vi "SubGenCodeRobot.vi"(8 "Edge Right Side":cluster{cluster{"Xrn":dbl, "Yrn":dbl}}[](array[cluster]), 11 "Edge Left Side":cluster{cluster{"Xln":dbl, "Yln":dbl}}[](array[cluster])) -> (3 "Source CODE Robot":string)   [LabVIEW 2015]
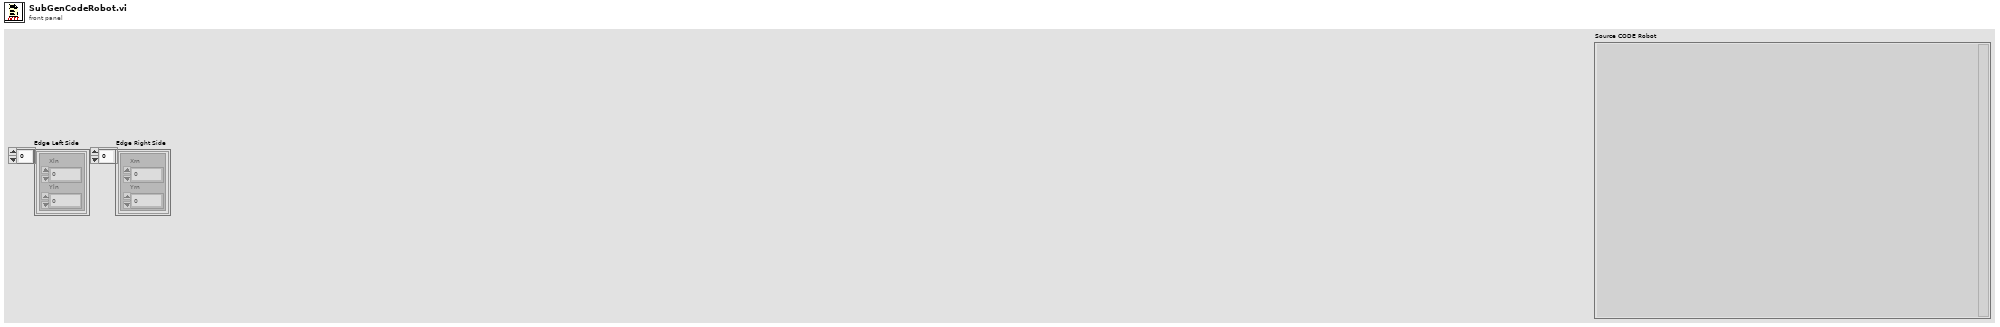
[diagram p1: front panel]
types:
  T1 = enum16{"open", "replace", "create", "open or create", "replace or create", "replace or create with confirmation"}
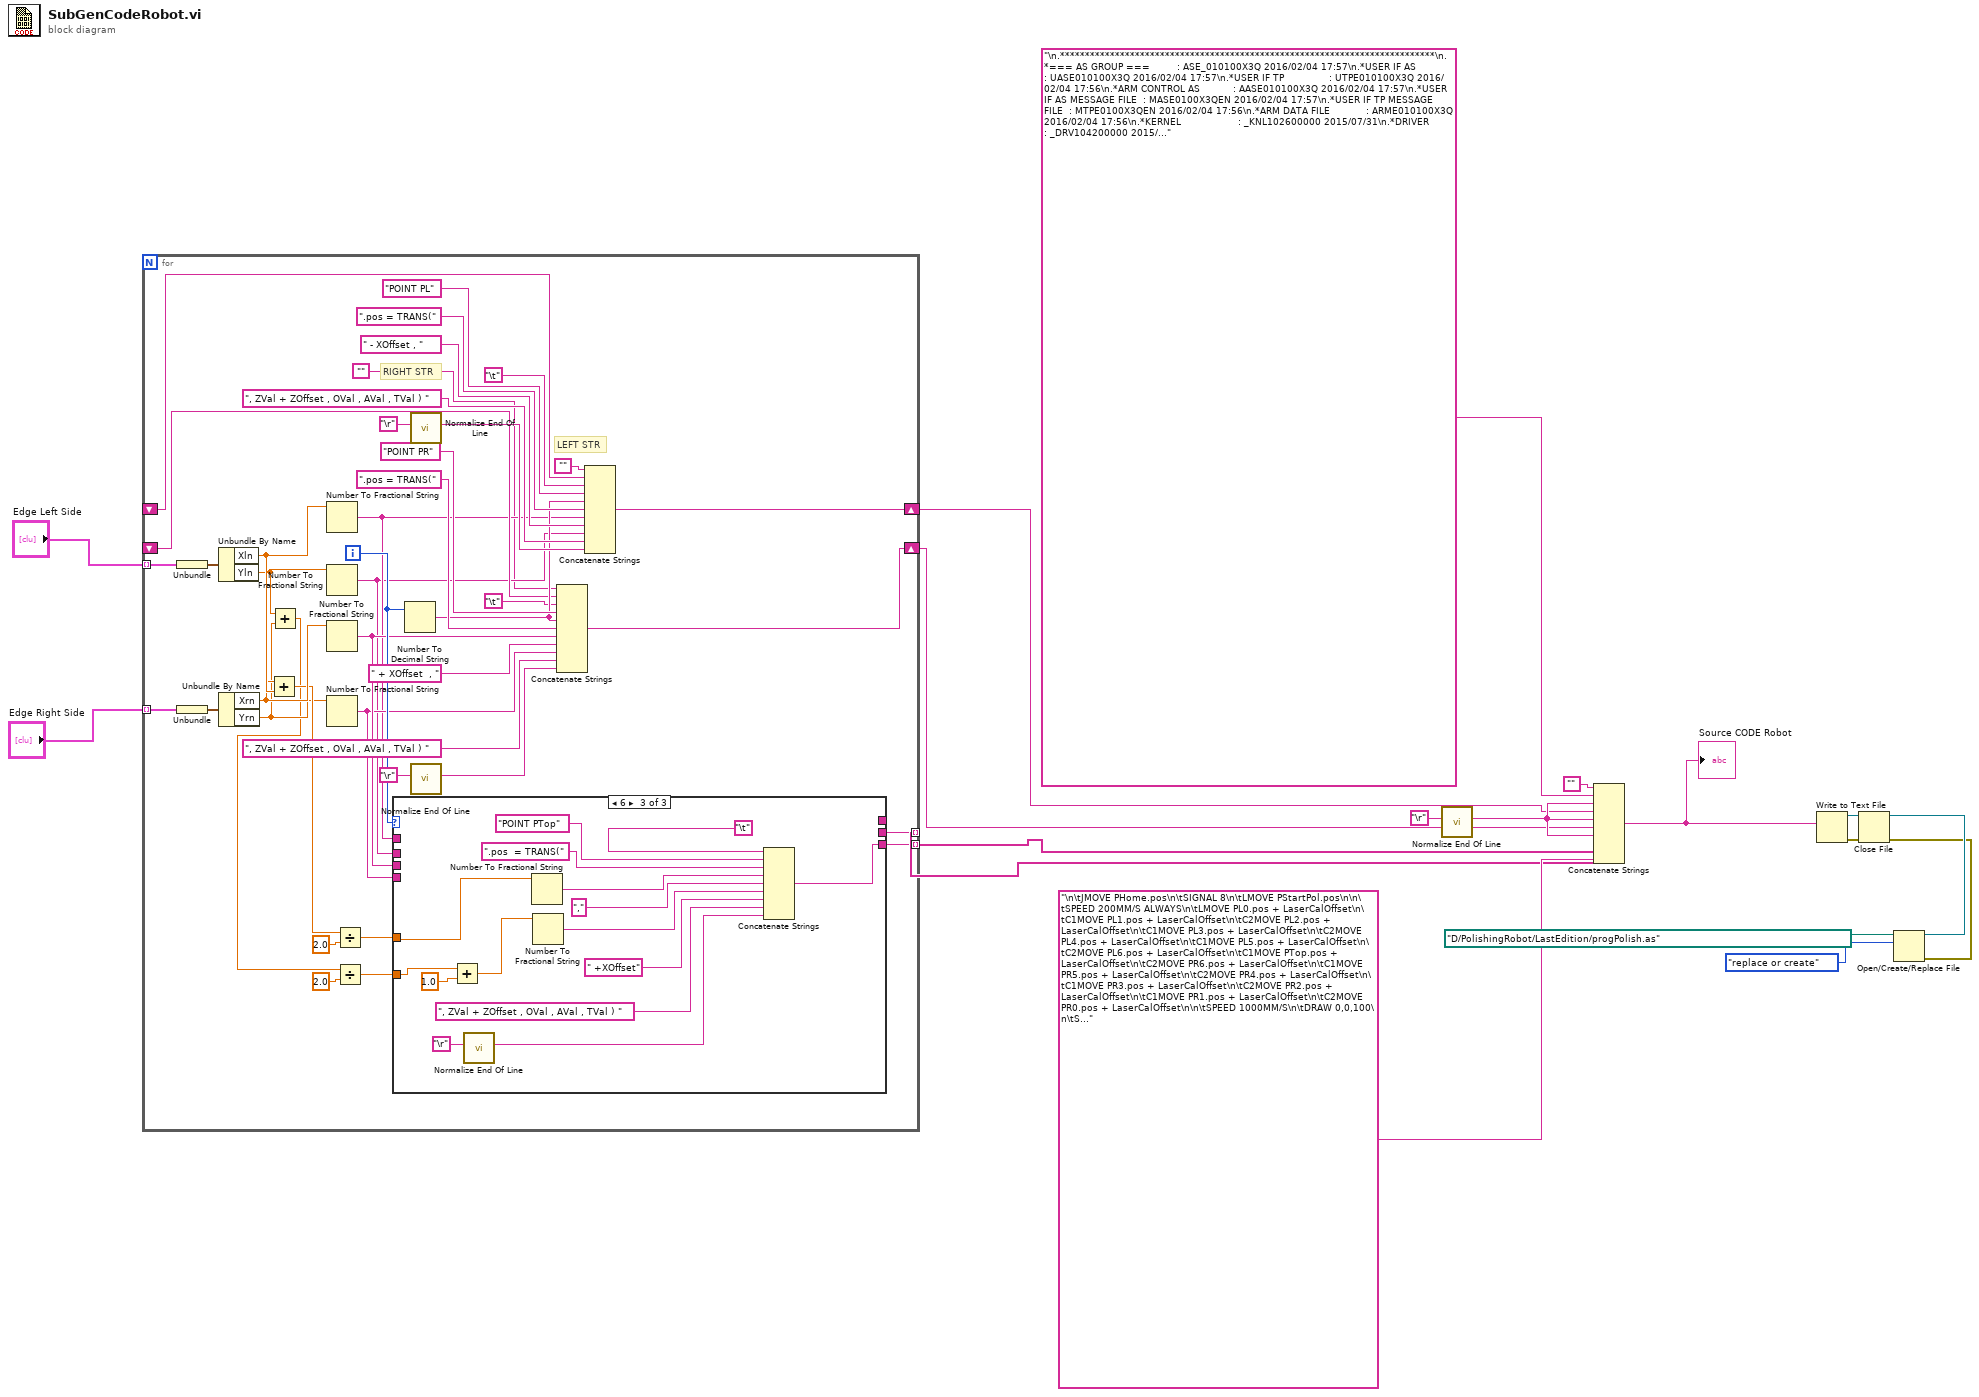
[diagram p0: block diagram]
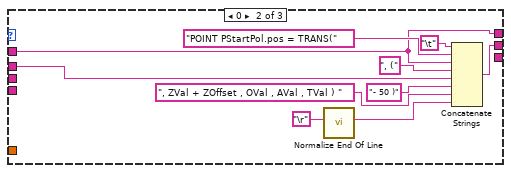
[diagram p3: hidden frame]
diagram:
  n1 = for {
    tunnel: "Edge Left Side" -> [w58] mode=indexing
    tunnel: "Edge Right Side" -> [w47] mode=indexing
    shift-right: [w43] -> w2
    shift-left: _ -> [w41]
    shift-right: [w42] -> w1
    shift-left: _ -> [w40]
    tunnel: [w34] -> w4 mode=indexing
    tunnel: [w33] -> w3 mode=indexing
    i -> [w37]
    # "RIGHT STR"
    # "LEFT STR"
    n2 = Unbundle(w58) -> (w57:cluster{"Xln":dbl, "Yln":dbl})
    n3 = Unbundle(w47) -> (w51:cluster{"Xrn":dbl, "Yrn":dbl})
    n4 = Unbundle By Name(w57) -> ("Xln"=w27:dbl, "Yln"=w23:dbl)
    n5 = Unbundle By Name(w51) -> ("Xrn"=w26:dbl, "Yrn"=w22:dbl)
    n6 = Add(x=w26, y=w27) -> (x+y=w25:dbl)
    n7 = Add(x=w23, y=w22) -> (x+y=w20:dbl)
    n8 = Number To Fractional String(number=w27) -> (F-format string=w32:string)  [unwired: 3 in]
    n9 = Number To Fractional String(number=w23) -> (F-format string=w31:string)  [unwired: 3 in]
    n10 = Number To Fractional String(number=w26) -> (F-format string=w36:string)  [unwired: 3 in]
    n11 = Number To Fractional String(number=w22) -> (F-format string=w35:string)  [unwired: 3 in]
    n12 = Divide(x=w25, y=2.0) -> (x/y=w24:dbl)
    n13 = Divide(x=w20, y=2.0) -> (x/y=w19:dbl)
    n14 = case shown="6" w37 {
      tunnel: w36 -> [_ _ _]
      tunnel: w35 -> [_ _ _]
      tunnel: [_ w63 _] -> w34
      tunnel: [_ _ w71] -> w33
      tunnel: [_ w62 _] -> _
      tunnel: w32 -> [_ w62 _]
      tunnel: w31 -> [_ w61 _]
      tunnel: w24 -> [_ _ w81]
      tunnel: w19 -> [_ _ w78]
      frame 99, Default {
      }
      frame 0 {
        n15 = call <vilib>:"Normalize End Of Line.vi"("string in"="\r") -> ("string out"=w64:string)  [unwired: 7 in]
        n16 = Concatenate Strings("\t", "POINT PStartPol.pos = TRANS(" ("string"), w62, ", (" ("string"), w61, "- 50 )" ("string"), ", ZVal + ZOffset , OVal , AVal , TVal ) " ("string"), w64) -> (w63:string)
      }
      frame 6 {
        n17 = Add(x=w78, y=1.0) -> (x+y=w76:dbl)
        n18 = call <vilib>:"Normalize End Of Line.vi"("string in"="\r") -> ("string out"=w72:string)  [unwired: 7 in]
        n19 = Number To Fractional String(number=w81) -> (F-format string=w80:string)  [unwired: 3 in]
        n20 = Number To Fractional String(number=w76) -> (F-format string=w75:string)  [unwired: 3 in]
        n21 = Concatenate Strings("\t", "POINT PTop" ("string"), ".pos  = TRANS(" ("string"), w80, "," ("string"), w75, " +XOffset" ("string"), ", ZVal + ZOffset , OVal , AVal , TVal ) " ("string"), w72) -> (w71:string)
      }
    }
    n22 = Number To Decimal String(number=w37) -> (decimal integer string=w46:string)  [unwired: 1 in]
    n23 = call <vilib>:"Normalize End Of Line.vi"("string in"="\r") -> ("string out"=w54:string)  [unwired: 7 in]
    n24 = call <vilib>:"Normalize End Of Line.vi"("string in"="\r") -> ("string out"=w48:string)  [unwired: 7 in]
    n25 = Concatenate Strings("", w40, "\t", "POINT PR" ("string"), w46, ".pos = TRANS(" ("string"), w36, " + XOffset  , " ("string"), w35, ", ZVal + ZOffset , OVal , AVal , TVal ) " ("string"), w48) -> (w42:string)
    n26 = Concatenate Strings("", w41, "\t", "POINT PL" ("string"), w46, ".pos = TRANS(" ("string"), w32, " - XOffset , " ("string"), w31, ", ZVal + ZOffset , OVal , AVal , TVal ) " ("string"), w54) -> (w43:string)
  }
  n27 = call <vilib>:"Normalize End Of Line.vi"("string in"="\r") -> ("string out"=w7:string)  [unwired: 7 in]
  n28 = Concatenate Strings("", "\n.***************************************************************************\n.*=== AS GROUP ===         : ASE_010100X3Q 2016/02/04 17:57\n.*USER IF AS               : UASE010100X3Q 2016/02/04 17:57\n.*USER IF TP               : UTPE010100X3Q 2016/02/04 17:56\n.*ARM CONTROL AS           : AASE010100X3Q 2016/02/04 17:57\n.*USER IF AS MESSAGE FILE  : MASE0100X3QEN 2016/02/04 17:57\n.*USER IF TP MESSAGE FILE  : MTPE0100X3QEN 2016/02/04 17:56\n.*ARM DATA FILE            : ARME010100X3Q 2016/02/04 17:56\n.*KERNEL                   : _KNL102600000 2015/07/31\n.*DRIVER                   : _DRV104200000 2015/01/30\n.*RFS                      : _RFS100800100 2012/07/27\n.*=== SERVO GROUP ===      : SVE_08000004H 2016/06/29 22:46\n.*ARM CONTROL SERVO        : ASVE08000004H 2016/06/29 22:44\n.*SRV DATA FILE            : ASPE08000004H 2016/06/29 22:44\n.*ARM CONTROL SERVO FPGA   : ASFE08000000A 2015/04/01 09:29\n.*\n.*Cpu board type           : 1VA\n.*=== WEB SERVER ===       : WBE_000000005\n.*   [Shipment setting data]\n.*There is no Shipment setting data.\n.***************************************************************************\n.NETCONF     192.168.0.2,\"timesys-\",255.255.255.0,192.168.0.1,0.0.0.0,0.0.0.0,\" \"\n.NETCONF2     192.168.11.2,255.255.255.0,0.0.0.0\n\n\n.PROGRAM GoHome\n\tOVal\t\t= 90\n\tAVal\t\t= 90\n\tTVal\t\t= -90\n\tPOINT PHome.pos = #[0.0, -35.0, -125.0, 0.0, 20.0, 0.0]\n\tJMOVE PHome.pos\n\tSIGNAL -8\n\tSTOP\n.END\n\n\n.PROGRAM PolishV1\n\tXOffset = 1\n\tZOffset = 0\n\tZVal    = 280\n\tOVal\t\t= 90\n\tAVal\t\t= 90\n\tTVal\t\t= -90\n\n\t; POINT LaserCalOffset  = TRANS(-54,2,0,0,0,0)\n\tPOINT LaserCalOffset  \t= TRANS(0,0,0,0,0,0)\n\tPOINT PHome.pos \t\t\t\t= #[0.0, -35.0, -125.0, 0.0, 20.0, 0.0]\n", w7, w2, w7, w1, w7, w4, w3, "\n\tJMOVE PHome.pos\n\tSIGNAL 8\n\tLMOVE PStartPol.pos\n\n\tSPEED 200MM/S ALWAYS\n\tLMOVE PL0.pos + LaserCalOffset\n\tC1MOVE PL1.pos + LaserCalOffset\n\tC2MOVE PL2.pos + LaserCalOffset\n\tC1MOVE PL3.pos + LaserCalOffset\n\tC2MOVE PL4.pos + LaserCalOffset\n\tC1MOVE PL5.pos + LaserCalOffset\n\tC2MOVE PL6.pos + LaserCalOffset\n\tC1MOVE PTop.pos + LaserCalOffset\n\tC2MOVE PR6.pos + LaserCalOffset\n\tC1MOVE PR5.pos + LaserCalOffset\n\tC2MOVE PR4.pos + LaserCalOffset\n\tC1MOVE PR3.pos + LaserCalOffset\n\tC2MOVE PR2.pos + LaserCalOffset\n\tC1MOVE PR1.pos + LaserCalOffset\n\tC2MOVE PR0.pos + LaserCalOffset\n\n\tSPEED 1000MM/S\n\tDRAW 0,0,100\n\tSIGNAL -8\n\tSPEED 2000MM/S\n\tJMOVE PHome.pos\n\n\tSTOP\n.END") -> (w11:string)
  "Source CODE Robot" <- w11
  n29 = Open/Create/Replace File(file path (use dialog)=path "D:/PolishingRobot/LastEdition/progPolish.as", operation (0:open)=T1."replace or create") -> (refnum out=w12:refnum<file>, error out=w10:errorcluster)  [unwired: 4 in, 1 out]
  n30 = Write to Text File(file (use dialog)=w12, text=w11, error in=w10) -> (refnum out=w14:refnum<file>, error out=w15:errorcluster)  [unwired: 1 in, 1 out]
  n31 = Close File(refnum=w14, error in=w15) -> ()  [unwired: 2 out]
